vi "937APressure.vi"(0 "VISA resource name":refnum<visa-resource-name>="COM1", 1 "error in (no error)":errorcluster) -> (2 "VISA resource name out":refnum<visa-resource-name>, 3 "Hi Spect":string, 4 "Lo Spect":string, 5 "error out":errorcluster)   [LabVIEW 2014]
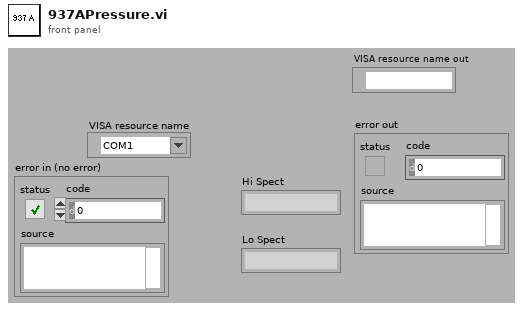
[diagram p1: front panel]
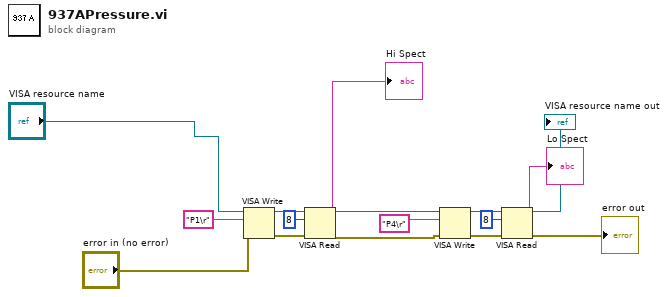
[diagram p0: block diagram]
diagram:
  n1 = VISA Write(VISA resource name="VISA resource name", write buffer="P1\r", error in (no error)="error in (no error)") -> (VISA resource name out=w14:refnum<visa-resource-name>, error out=w8:errorcluster)  [unwired: 1 out]
  n2 = VISA Read(VISA resource name=w14, byte count=u32 8, error in (no error)=w8) -> (VISA resource name out=w6:refnum<visa-resource-name>, read buffer=→"Hi Spect":string, error out=w5:errorcluster)  [unwired: 1 out]
  n3 = VISA Write(VISA resource name=w6, write buffer="P4\r", error in (no error)=w5) -> (VISA resource name out=w12:refnum<visa-resource-name>, error out=w9:errorcluster)  [unwired: 1 out]
  n4 = VISA Read(VISA resource name=w12, byte count=u32 8, error in (no error)=w9) -> (VISA resource name out=→"VISA resource name out":refnum<visa-resource-name>, read buffer=→"Lo Spect":string, error out=→"error out":errorcluster)  [unwired: 1 out]
